vi "DSF.Engine.Transceiver Loader.Find Packed Libraries.vi"(8 "error in (no error)":errorcluster, 11 "Transceiver Loader in":refnum<class "DSF.Engine.Transceiver Loader.lvclass">) -> (0 "error out":errorcluster, 2 "packed library paths":path[](array[path]), 3 "Transceiver Loader out":refnum<class "DSF.Engine.Transceiver Loader.lvclass">)   [LabVIEW 2017, in "DSF.Engine.lvlib" / "DSF.Engine.Transceiver Loader.lvclass"]
uses:
  DSF.Engine.Transceiver Loader.lvclass
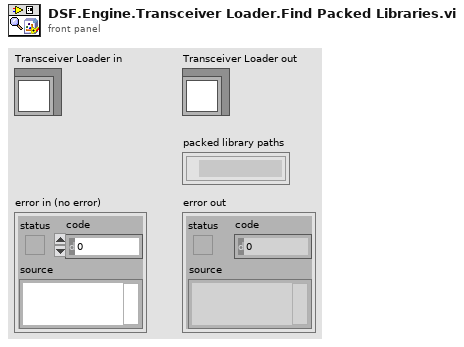
[diagram p1: front panel]
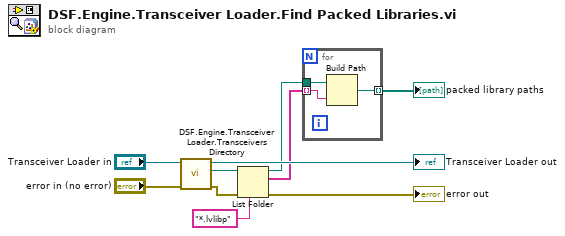
[diagram p0: block diagram]
diagram:
  n1 = call "DSF.Engine.Transceiver Loader.Transceivers Directory.vi"("error in (no error)"="error in (no error)", "Transceiver Loader in"="Transceiver Loader in") -> ("error out"=w4:errorcluster, "transceivers directory"=w8:path, "Transceiver Loader out"=→"Transceiver Loader out":refnum<class "DSF.Engine.Transceiver Loader.lvclass">)  [unwired: 7 in]
  n2 = List Folder(path=w8, pattern="*.lvlibp", error in=w4) -> (path out=w6:path, filenames=w2:string[], error out=→"error out":errorcluster)  [unwired: 1 in, 1 out]
  n3 = for {
    tunnel: w2 -> [w12] mode=indexing
    tunnel: w6 -> [w13]
    tunnel: [w11] -> w3 mode=indexing
    n4 = Build Path(base path=w13, name or relative path=w12) -> (appended path=w11:path)
  }
  "packed library paths" <- w3
